vi "Append to command queue.vi"(3 "Name (CommandQueue)":string="CommandQueue", 5 "Clear Queue (F)":bool, 7 "Position":enum16{"End", "Beginning"}(ring), 8 "error in (no error)":errorcluster, 9 "Command Array":string[](array[string]), 10 "Single command":string, 11 "Error Ref (not required)":refnum<vi>) -> (0 "error out":errorcluster)   [LabVIEW 2016]
doc: "Appends a command, or an array of commands, to the command queue 'CommandQueue\". If you wish for this VI to report error, pass a Refnum to an error indicator/control. You may choose to append the commands at the beginning of the queue, causing them to be executed before any other commands in the queue. Use the \"position\" input for this. Default is End."
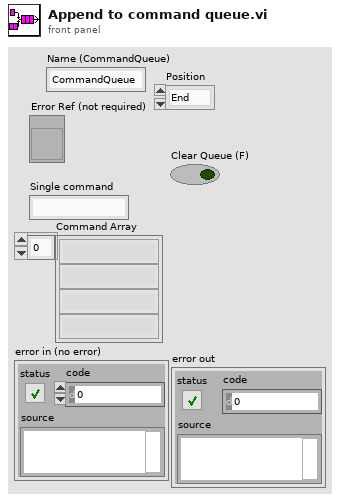
[diagram p1: front panel]
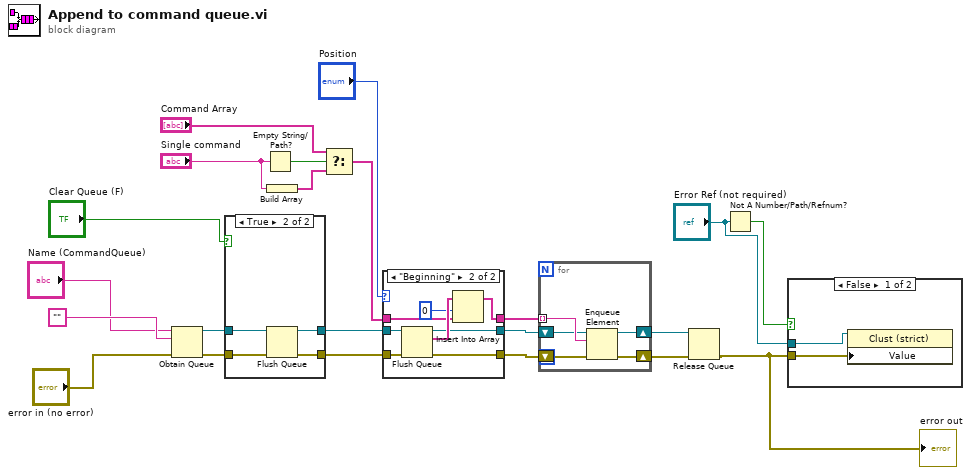
[diagram p0: block diagram]
diagram:
  n1 = Obtain Queue(name (unnamed)="Name (CommandQueue)", element data type="", error in (no error)="error in (no error)") -> (queue out=w8:refnum<queue>, error out=w7:errorcluster)  [unwired: 2 in, 1 out]
  n2 = case shown="True" "Clear Queue (F)" {
    tunnel: w8 -> [w24 w28]
    tunnel: w7 -> [w23 w27]
    tunnel: [w24 w26] -> w5
    tunnel: [w23 w25] -> w6
    frame False {
    }
    frame True {
      n3 = Flush Queue(queue=w28, error in (no error)=w27) -> (queue out=w26:refnum<queue>, error out=w25:errorcluster)  [unwired: 1 out]
    }
  }
  n4 = Empty String/Path?(string/path="Single command") -> (empty?=w19:bool)
  n5 = Build Array("Single command") -> (w17:string[])
  n6 = Select(t="Command Array", s=w19, f=w17) -> (s? t:f=w13:string[])
  n7 = case shown="\"Beginning\"" "Position" {
    tunnel: w5 -> [w30 w39]
    tunnel: w6 -> [w29 w38]
    tunnel: w13 -> [w31 w36]
    tunnel: [w31 w35] -> w12
    tunnel: [w29 w33] -> w11
    tunnel: [w30 w32] -> w10
    frame "End", Default {
    }
    frame "Beginning" {
      n8 = Flush Queue(queue=w39, error in (no error)=w38) -> (queue out=w32:refnum<queue>, remaining elements=w37:string[], error out=w33:errorcluster)
      n9 = Insert Into Array(array=w37, index=0, new element=w36) -> (w35:string[])
    }
  }
  n10 = for {
    tunnel: w12 -> [w43] mode=indexing
    shift-right: [w44] -> w3
    shift-left: w11 -> [w42]
    shift-right: [w41] -> w2
    shift-left: w10 -> [w40]
    n11 = Enqueue Element(queue=w40, element=w43, error in (no error)=w42) -> (queue out=w41:refnum<queue>, error out=w44:errorcluster)  [unwired: 1 in, 1 out]
  }
  n12 = Release Queue(queue=w2, error in (no error)=w3) -> (error out=w1:errorcluster)  [unwired: 1 in, 2 out]
  "error out" <- w1
  n13 = Not A Number/Path/Refnum?(number/path/refnum="Error Ref (not required)") -> (NaN/Path/Refnum?=w14:bool)
  n14 = case shown="False" w14 {
    tunnel: w1 -> [w46 _]
    tunnel: "Error Ref (not required)" -> [w45 _]
    frame False {
      n15 = property class="Clust (strict)"(reference=w45, "Value"=w46) -> ()  [unwired: 1 in, 2 out]
    }
    frame True {
    }
  }
